vi "Format Device Configuration Log.vi"(8 "error in (no error)":errorcluster, 11 "Instrument.Lockin in":refnum<class "Instrument.Lockin.lvclass">) -> (0 "error out":errorcluster, 1 "Device Configuration":T1[](array[typedef]), 2 "Log Paths":string, 3 "Instrument.Lockin out":refnum<class "Instrument.Lockin.lvclass">, 4 "Times":timestamp[](array[timestamp]))   [LabVIEW 2019, in "Instrument.Lockin.lvlib" / "Instrument.Lockin.lvclass"]
uses:
  Instrument.Lockin.lvclass
  Typedefs/Lockin.LogConfiguration.Devices--Cluster.ctl
  Instrument.Lockin.lvclass/Instrument.Lockin.ctl
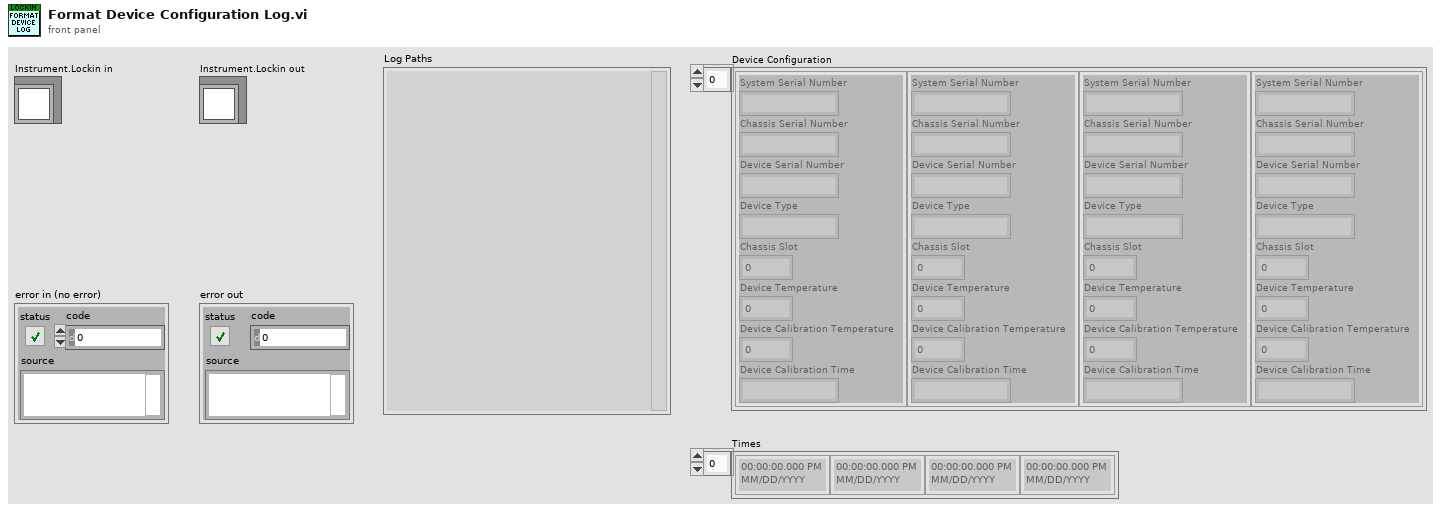
[diagram p1: front panel]
types:
  T1 = typedef "Instrument.Lockin.lvlib/Instrument.Lockin.lvclass/Lockin.LogConfiguration.Devices--Cluster.ctl" = cluster{"System Serial Number":string, "Chassis Serial Number":string, "Device Serial Number":string, "Device Type":string, "Chassis Slot":i32, "Device Temperature":dbl, "Device Calibration Temperature":dbl, "Device Calibration Time":string}
  T2 = typedef "Instrument.Lockin.lvlib/Instrument.DAQ.lvclass/DeviceInfo--Cluster.ctl" = cluster{"DeviceName":string, "DevIsSimulated":bool, "DeviceSerialNumber":string, "ProductType":string, "ProductCategory":i32, "ProductNumber":u32, "ChassisNumber":u32, "SlotNumber":u32, "ChassisName":string, "ChassisSerialNumber":string, "DevTemp":dbl, "SelfCal.LastDate/Time":string, "SelfCal.LastTemp":dbl, "calibration due?":bool}
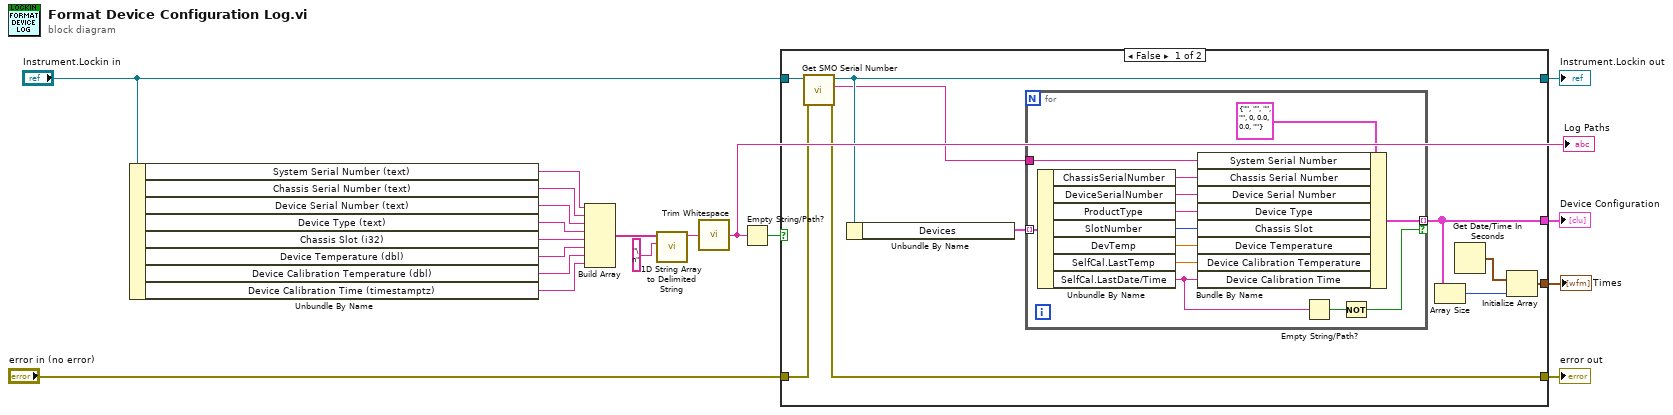
[diagram p0: block diagram]
diagram:
  n1 = Unbundle By Name("Instrument.Lockin in") -> ("System Serial Number (text)"=w12:string, "Chassis Serial Number (text)"=w11:string, "Device Serial Number (text)"=w10:string, "Device Type (text)"=w9:string, "Chassis Slot (i32)"=w8:string, "Device Temperature (dbl)"=w7:string, "Device Calibration Temperature (dbl)"=w6:string, "Device Calibration Time (timestamptz)"=w5:string)
  n2 = Build Array(w12, w11, w10, w9, w8, w7, w6, w5) -> (w3:string[])
  n3 = call <vilib>:"1D String Array to Delimited String.vi"("delimiter"="\n", "string array"=w3) -> ("delimited string"=w14:string)  [unwired: 9 in]
  n4 = call <vilib>:"Trim Whitespace.vi"("string"=w14) -> ("trimmed string"=w13:string)  [unwired: 1 in]
  "Log Paths" <- w13
  n5 = Empty String/Path?(string/path=w13) -> (empty?=w2:bool)
  n6 = case shown="False" w2 {
    tunnel: [w29 w43] -> w19
    tunnel: "error in (no error)" -> [w26 w44]
    tunnel: [w25 w44] -> w17
    tunnel: [w22 _] -> w16
    tunnel: "Instrument.Lockin in" -> [w24 w43]
    tunnel: [w21 _] -> w1
    frame False {
      n7 = call-dynamic "Get SMO Serial Number.vi"("error in (no error)"=w26, "Instrument.Lockin in"=w24) -> ("error out"=w25:errorcluster, "Serial Number"=w28:string, "Instrument.Lockin out"=w29:refnum<class "Instrument.Lockin.lvclass">)  [unwired: 7 in]
      n8 = Unbundle By Name(w29) -> ("Devices"=w27:T2[])
      n9 = for {
        tunnel: [w42] -> w22 mode=indexing if=w30
        tunnel: w28 -> [w40]
        tunnel: w27 -> [w41] mode=indexing
        n10 = Unbundle By Name(w41) -> ("ChassisSerialNumber"=w39:string, "DeviceSerialNumber"=w38:string, "ProductType"=w37:string, "SlotNumber"=w36:u32, "DevTemp"=w34:dbl, "SelfCal.LastTemp"=w35:dbl, "SelfCal.LastDate/Time"=w31:string)
        n11 = Bundle By Name(cluster=T1 {"System Serial Number"="", "Chassis Serial Number"="", "Device Serial Number"="", "Device Type"="", "Chassis Slot"=0, "Device Temperature"=0.0, "Device Calibration Temperature"=0.0, "Device Calibration Time"=""} ("Device Configuration"), "System Serial Number"=w40, "Chassis Serial Number"=w39, "Device Serial Number"=w38, "Device Type"=w37, "Chassis Slot"=w36, "Device Temperature"=w34, "Device Calibration Temperature"=w35, "Device Calibration Time"=w31) -> (w42:T1)
        n12 = Empty String/Path?(string/path=w31) -> (empty?=w32:bool)
        n13 = Not(x=w32) -> (.not. x?=w30:bool)
      }
      n14 = Array Size(array=w22) -> (size(s)=w20:i32)
      n15 = Get Date/Time In Seconds() -> (seconds since 1Jan1904=w23:timestamp)
      n16 = Initialize Array(w23, w20) -> (w21:timestamp[])
    }
    frame True {
    }
  }
  "Instrument.Lockin out" <- w19
  "error out" <- w17
  "Device Configuration" <- w16
  "Times" <- w1
